vi "CANcoder_open.vi"(10 "CANbus Name":string="rio", 11 "Device ID":u8) -> (3 "DeviceReference 2":T1)   [LabVIEW 2020]
uses:
  DeviceReference.ctl
  <userlib>/CTRE_PhoenixTools/CTRE_PhoenixTools.lvlib
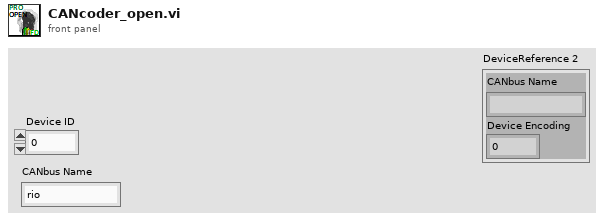
[diagram p1: front panel]
types:
  T1 = typedef "DeviceReference.ctl" = cluster{"CANbus Name":string, "Device Encoding":u32}
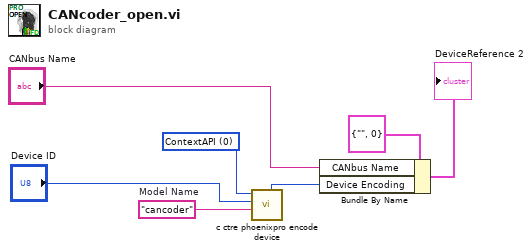
[diagram p0: block diagram]
diagram:
  w4 = u32 0 items=["ContextAPI", "ContextDiagServer"] ("context")
  w2 = "cancoder"  # Model Name
  n1 = call <userlib>:"c ctre phoenixpro encode device.vi"("model"=w2, "deviceId"="Device ID", "context"=w4) -> ("deviceEncoding out"=w1:u32)  [unwired: 6 in, 2 out]
  n2 = Bundle By Name(cluster=T1 {"CANbus Name"="", "Device Encoding"=0} ("DeviceReference"), "CANbus Name"="CANbus Name", "Device Encoding"=w1) -> (→"DeviceReference 2":T1)
